vi "Find Diamonds.vi"(10 "Filtered Targets":T4[](array[typedef]), 11 "Lines":T1[][](array[typedef])) -> (3 "Diamond Targets":T5[](array[typedef]))   [LabVIEW 2011]
uses:
  Diamond Target Output.ctl
  Rectangle Position.ctl
  Target.ctl
  Line.ctl
  Direction.ctl
  Line Confidence.ctl
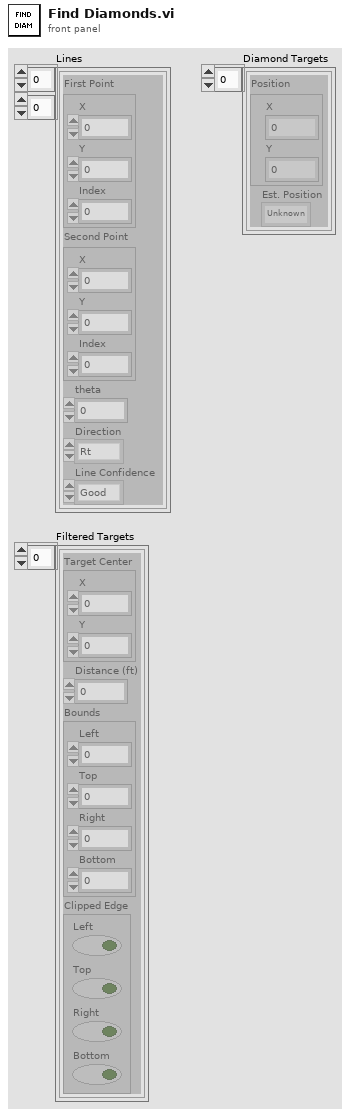
[diagram p1: front panel]
types:
  T1 = typedef "Line.ctl" = cluster{"First Point":cluster{"X":dbl, "Y":dbl, "Index":dbl}, "Second Point":cluster{"X":dbl, "Y":dbl, "Index":dbl}, "theta":dbl, "Direction":T2, "Line Confidence":T3}
  T2 = typedef "Direction.ctl" = enum16{"Rt", "Rt-Up", "Up", "Lt-Up", "Lt", "Lt-Dn", "Dn", "Rt-Dn"}
  T3 = typedef "Line Confidence.ctl" = enum16{"Good", "Bad"}
  T4 = typedef "Target.ctl" = cluster{"Target Center":cluster{"X":dbl, "Y":dbl}, "Distance (ft)":dbl, "Bounds":cluster{"Left":dbl, "Top":dbl, "Right":dbl, "Bottom":dbl}, "Clipped Edge":cluster{"Left":bool, "Top":bool, "Right":bool, "Bottom":bool}}
  T5 = typedef "Diamond Target Output.ctl" = cluster{"Position":cluster{"X":dbl, "Y":dbl}, "Est. Position":T6}
  T6 = typedef "Rectangle Position.ctl" = enum16{"Unknown", "Top", "Right", "Left", "Bottom"}
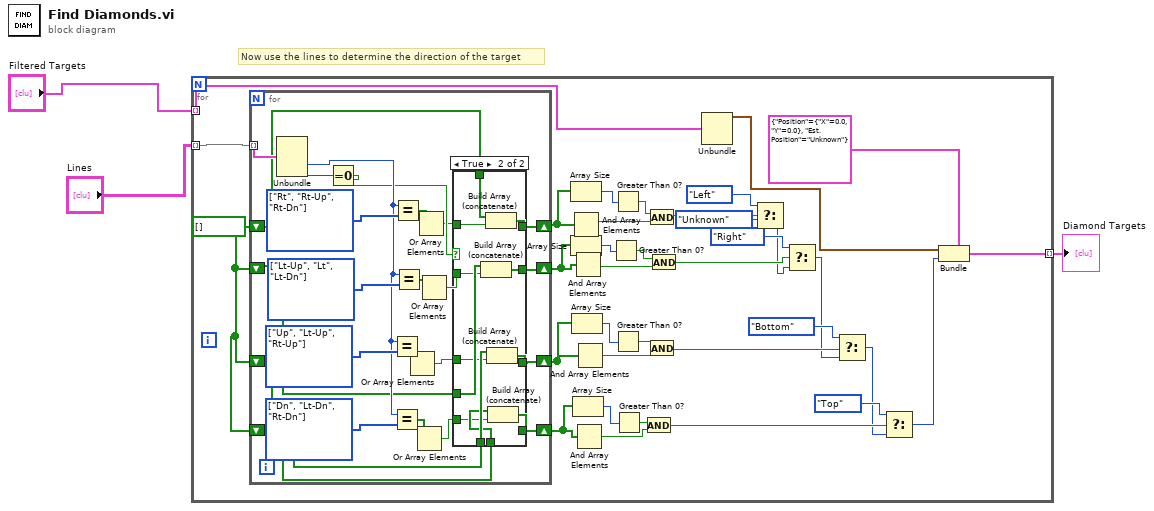
[diagram p0: block diagram]
diagram:
  # "Now use the lines to determine the direction of the target"
  n1 = for {
    tunnel: "Lines" -> [w38] mode=indexing
    tunnel: "Filtered Targets" -> [w8] mode=indexing
    tunnel: [w4] -> w3 mode=indexing
    w37 = bool[] []
    n2 = for {
      tunnel: w38 -> [w62] mode=indexing
      shift-right: [w54] -> w32
      shift-left: w37 -> [w53]
      shift-right: [w52] -> w31
      shift-left: w37 -> [w51]
      shift-right: [w39] -> w30
      shift-left: w37 -> [w50]
      shift-right: [w49] -> w29
      shift-left: w37 -> [w48]
      w57 = T2[] [enum."Dn", enum."Lt-Dn", enum."Rt-Dn"] items=["Rt", "Rt-Up", "Up", "Lt-Up", "Lt", "Lt-Dn", "Dn", "Rt-Dn"]
      w58 = T2[] [enum."Up", enum."Lt-Up", enum."Rt-Up"] items=["Rt", "Rt-Up", "Up", "Lt-Up", "Lt", "Lt-Dn", "Dn", "Rt-Dn"]
      w59 = T2[] [enum."Lt-Up", enum."Lt", enum."Lt-Dn"] items=["Rt", "Rt-Up", "Up", "Lt-Up", "Lt", "Lt-Dn", "Dn", "Rt-Dn"]
      w60 = T2[] [enum."Rt", enum."Rt-Up", enum."Rt-Dn"] items=["Rt", "Rt-Up", "Up", "Lt-Up", "Lt", "Lt-Dn", "Dn", "Rt-Dn"]
      n3 = Unbundle(w62) -> ("Direction"=w56:T2, "Line Confidence"=w61:T3)  [unwired: 3 out]
      n4 = Equal To 0?(x=w61) -> (x = 0?=w55:bool)
      n5 = Equal?(x=w56, y=w58) -> (x = y?=w42:bool[])
      n6 = Equal?(x=w56, y=w57) -> (x = y?=w40:bool[])
      n7 = Equal?(x=w56, y=w60) -> (x = y?=w46:bool[])
      n8 = Equal?(x=w56, y=w59) -> (x = y?=w44:bool[])
      n9 = Or Array Elements(Boolean array=w42) -> (logical OR=w43:bool)
      n10 = Or Array Elements(Boolean array=w40) -> (logical OR=w41:bool)
      n11 = Or Array Elements(Boolean array=w46) -> (logical OR=w47:bool)
      n12 = Or Array Elements(Boolean array=w44) -> (logical OR=w45:bool)
      n13 = case shown="True" w55 {
        tunnel: [w66 w78] -> w54
        tunnel: w53 -> [w66 w77]
        tunnel: w47 -> [_ w76]
        tunnel: [w65 w75] -> w52
        tunnel: w51 -> [w65 w74]
        tunnel: w45 -> [_ w73]
        tunnel: [w64 w72] -> w39
        tunnel: w50 -> [w64 w71]
        tunnel: w43 -> [_ w70]
        tunnel: [w63 w69] -> w49
        tunnel: w48 -> [w63 w68]
        tunnel: w41 -> [_ w67]
        frame False {
        }
        frame True {
          n14 = Build Array (concatenate)(w74, w73) -> (w75:bool[])
          n15 = Build Array (concatenate)(w77, w76) -> (w78:bool[])
          n16 = Build Array (concatenate)(w71, w70) -> (w72:bool[])
          n17 = Build Array (concatenate)(w68, w67) -> (w69:bool[])
        }
      }
    }
    n18 = Array Size(array=w32) -> (size(s)=w27:i32)
    n19 = And Array Elements(Boolean array=w32) -> (logical AND=w36:bool)
    n20 = Array Size(array=w31) -> (size(s)=w25:i32)
    n21 = Array Size(array=w30) -> (size(s)=w23:i32)
    n22 = And Array Elements(Boolean array=w31) -> (logical AND=w35:bool)
    n23 = Array Size(array=w29) -> (size(s)=w22:i32)
    n24 = And Array Elements(Boolean array=w29) -> (logical AND=w33:bool)
    n25 = And Array Elements(Boolean array=w30) -> (logical AND=w34:bool)
    n26 = Greater Than 0?(x=w25) -> (x > 0?=w26:bool)
    n27 = Greater Than 0?(x=w27) -> (x > 0?=w28:bool)
    n28 = Greater Than 0?(x=w23) -> (x > 0?=w24:bool)
    n29 = Greater Than 0?(x=w22) -> (x > 0?=w21:bool)
    n30 = And(x=w21, y=w33) -> (x .and. y?=w14:bool)
    n31 = And(x=w28, y=w36) -> (x .and. y?=w20:bool)
    n32 = And(x=w24, y=w34) -> (x .and. y?=w16:bool)
    n33 = And(x=w26, y=w35) -> (x .and. y?=w18:bool)
    n34 = Unbundle(w8) -> ("Target Center"=w6:cluster{"X":dbl, "Y":dbl})  [unwired: 3 out]
    n35 = Select(t=Rectangle_Position."Left" ("Rectangle Position"), s=w20, f=Rectangle_Position."Unknown") -> (s? t:f=w11:T6)
    n36 = Select(t=Rectangle_Position."Right" ("Rectangle Position"), s=w18, f=w11) -> (s? t:f=w12:T6)
    n37 = Select(t=Rectangle_Position."Bottom" ("Rectangle Position"), s=w16, f=w12) -> (s? t:f=w13:T6)
    n38 = Select(t=Rectangle_Position."Top" ("Rectangle Position"), s=w14, f=w13) -> (s? t:f=w5:T6)
    n39 = Bundle(cluster=T5 {"Position"={"X"=0.0, "Y"=0.0}, "Est. Position"=enum."Unknown"} ("Diamond Target Type"), "Position"=w6, "Est. Position"=w5) -> (w4:T5)
  }
  "Diamond Targets" <- w3
